vi "area of triangle (Sub VI) lab 4.vi"(9 "C":dbl, 10 "B":dbl, 11 "A":dbl) -> (2 "Area":dbl, 3 "S":dbl)   [LabVIEW 2016]
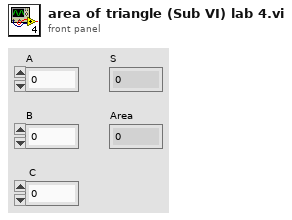
[diagram p1: front panel]
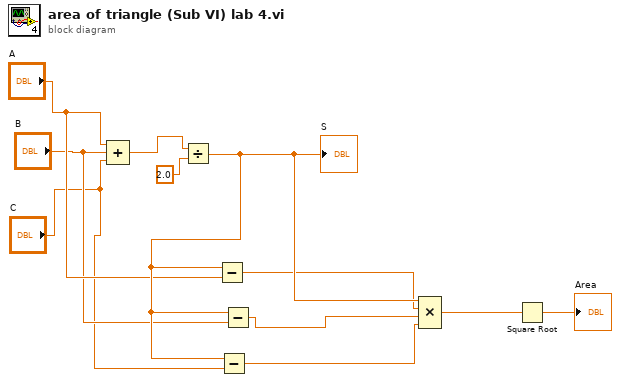
[diagram p0: block diagram]
diagram:
  n1 = Compound Arithmetic op=ADD("A", "B", "C") -> (w5:dbl)
  n2 = Divide(x=w5, y=2.0 ("x")) -> (x/y=w11:dbl)
  "S" <- w11
  n3 = Subtract(x=w11, y="A") -> (x-y=w10:dbl)
  n4 = Subtract(x=w11, y="C") -> (x-y=w8:dbl)
  n5 = Subtract(x=w11, y="B") -> (x-y=w9:dbl)
  n6 = Compound Arithmetic op=MULTIPLY(w11, w10, w9, w8) -> (w7:dbl)
  n7 = Square Root(x=w7) -> (sqrt(x)=→"Area":dbl)
